vi "Silhouette_Samples.vi"(8 "error in (no error)":errorcluster caption="entrée d'erreur (pas d'erreur)", 9 "labels":string[][](array[string]), 10 "X":string[][](array[string]), 11 "silhouette_samples":cluster{"metric":string}={"metric"="euclidean"}) -> (0 "error out":errorcluster caption="sortie d'erreur", 3 "Data":T1)   [LabVIEW 2020]
doc: "Compute the Silhouette Coefficient for each sample.\n\nThe Silhouette Coefficient is a measure of how well samples are clustered with samples that are similar to themselves. Clustering models with a high Silhouette Coefficient are said to be dense, where samples in the same cluster are similar to each other, and well separated, where samples in different clusters are not very similar to each other.\n\nThe Silhouette Coefficient is calculated using the mean intra-cluster distance (a) and the mean nearest-cluster distance (b) for each sample. The Silhouette Coefficient for a sample is (b - a) / max(a, b). Note that Silhouette Coefficient is only defined if number of labels is 2 <= n_labels <= n_samples - 1.\n\nThis function returns the Silhouette Coefficient for each sample.\n\nThe best value is 1 and the worst value is -1. Values near 0 indicate overlapping clusters.\n\n\n\nParameters : \n\n- X : array [n_samples_a, n_samples_a] if metric == “precomputed”, or, [n_samples_a, n_features] otherwise\nArray of pairwise distances between samples, or a feature array.\n\n- labels : array, shape = [n_samples]\nlabel values for each sample\n\n- metric : string, or callable\nThe metric to use when calculating distance between instances in a feature array. If metric is a string, it must be one of the options allowed by sklearn.metrics.pairwise.pairwise_distances. If X is the distance array itself, use “precomputed” as the metric. Precomputed distance matrices must have 0 along the diagonal.\n\nReturns : \n\n- silhouette : array, shape = [n_samples]\nSilhouette Coefficient for each samples."
uses:
  Silhouette_Samples.lvclass
panel:
  out "Silhouette_Samples.lvclass":refnum<class "Silhouette_Samples.lvclass">
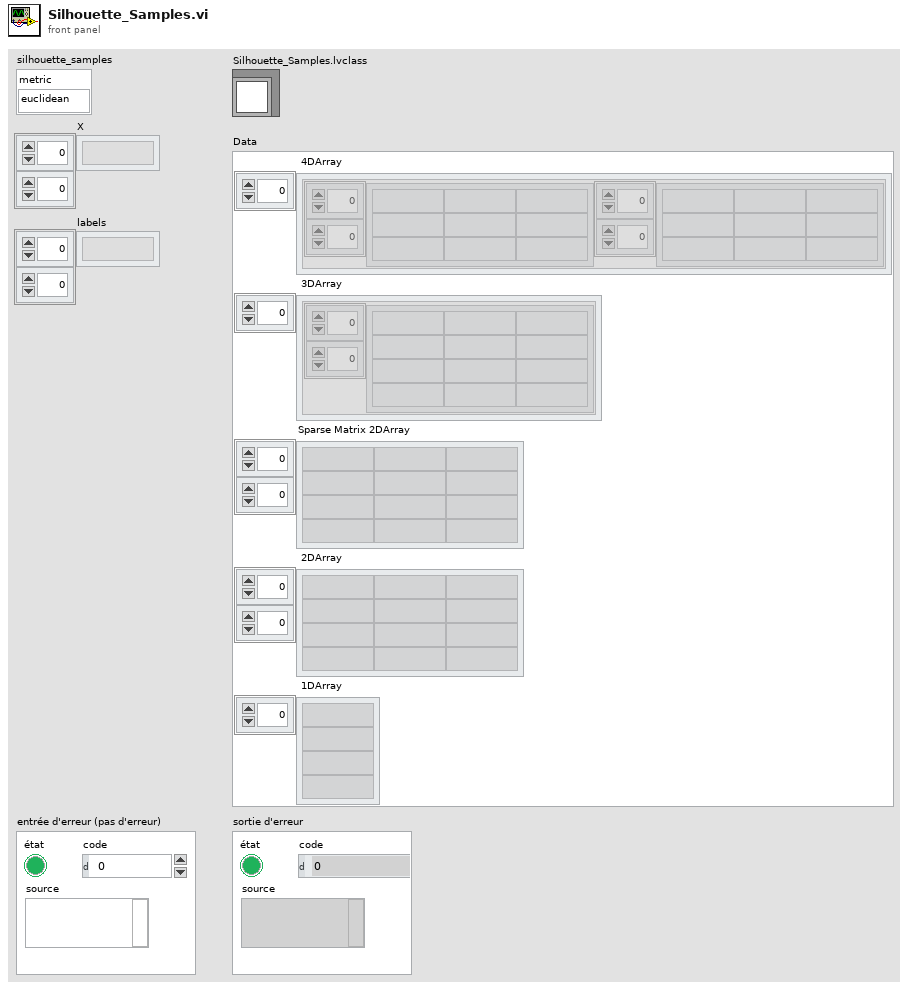
[diagram p1: front panel]
types:
  T1 = cluster{" 4DArray":cluster{"1":string[][], "2":string[][]}[], " 3DArray":cluster{"Tableau":string[][]}[], "Sparse Matrix 2DArray":string[][], " 2DArray":string[][], " 1DArray":string[]}
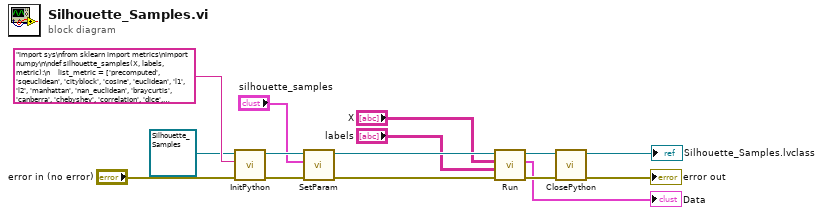
[diagram p0: block diagram]
diagram:
  n1 = call-dynamic "InitPython.vi"("error in (no error)"="error in (no error)", "Python Instruction"="import sys\nfrom sklearn import metrics\nimport numpy\n\ndef silhouette_samples(X, labels, metric):\n    list_metric = ['precomputed', 'sqeuclidean', 'cityblock', 'cosine', 'euclidean', 'l1', 'l2', 'manhattan', 'nan_euclidean', 'braycurtis', 'canberra', 'chebyshev', 'correlation', 'dice', 'hamming', 'jaccard', 'kulsinski', 'mahalanobis', 'minkowski', 'rogerstanimoto', 'russellrao', 'seuclidean', 'sokalmichener', 'sokalsneath', 'sqeuclidean', 'yule']\n    X = eval(X)\n    labels = eval(labels)\n    if metric not in list_metric:\n        metric = eval(metric) \n    try:\n        silhouette_samples = metrics.silhouette_samples(X, labels, metric)\n        silhouette_samples = silhouette_samples.tolist()\n        return str(silhouette_samples)\n    except:\n        erreur = sys.exc_info()\n        typerr = u\"%s\" % (erreur[0])\n        typerr = typerr[typerr.find(\"'\")+1:typerr.rfind(\"'\")]\n        msgerr = u\"%s\" % (erreur[1])\n        message = str('/!\\\\ {0} : {1}'. format(typerr,msgerr))\n        return message", "Scikit-learn en entrée"=refnum<class "Silhouette_Samples.lvclass"> refnum ("Silhouette_Samples.lvclass")) -> ("error out"=w8:errorcluster, "Scikit-learn en sortie"=w10:refnum<class "Silhouette_Samples.lvclass">)  [unwired: 7 in]
  n2 = call-dynamic "SetParam.vi"("error in (no error)"=w8, "silhouette_samples"="silhouette_samples", "Silhouette_Samples.lvclass"=w10) -> ("error out"=w6:errorcluster, "Silhouette_Samples.lvclass"=w7:refnum<class "Silhouette_Samples.lvclass">)  [unwired: 7 in]
  n3 = call-dynamic "Run.vi"("error in (no error)"=w6, "labels"="labels", "X"="X", "Silhouette_Samples.lvclass"=w7) -> ("error out"=w11:errorcluster, "Data"=→"Data":T1, "Silhouette_Samples.lvclass"=w12:refnum<class "Silhouette_Samples.lvclass">)  [unwired: 5 in]
  n4 = call-dynamic "ClosePython.vi"("error in (no error)"=w11, "Scikit-learn en entrée"=w12) -> ("error out"=→"error out":errorcluster, "Scikit-learn en sortie"=→"Silhouette_Samples.lvclass":refnum<class "Silhouette_Samples.lvclass">)  [unwired: 8 in]
